vi "Vision Research Phantom Series PhLV Progress.vi"(3 "Continue":bool, 5 "Error In (no error)":errorcluster, 7 "CallID":u32) -> (16 "pPercent":u32, 19 "Error Out":errorcluster)   [LabVIEW 2013, in "VRI.lvlib"]
doc: "PhCon.dll\n\nUse this to have a progress indicator (ex. when reading the stg from flash or saving a cine)\n\nPhLVProgress\nHRESULT PhLVProgress(UINT CallID, PUINT pPercent, BOOL Continue);\n\nParameters Description\nCallID (in) The call identifier (a number from 1 to 15), which was passed as a \n PROGRESSCALLBACK parameter in a time consuming function.\npPercent(out) The percentage of work done for the time consuming routine call, identified\n by CallID. \nContinue(in) Specifies if the function must continue.\n TRUE - to continue\n FALSE - to stop the function call, and force it to return.\nReturn HRESULT (0 = Ok)\nComments This function is used as a progress indicator for time-consuming functions.\n It is designed to work with environments which do not support function\n pointers (like LabVIEW).\n The time-consuming function call and the PhLVProgress call must be in \n different threads.\n In LabVIEW the time-consuming function call node must be set to Reentrant.\n All API calls that have a PROGRESSCALLBACK function pointer parameter\n accept a CallID in it. CallID is a UINT and it must be in the range [1, 15]. \n After calling such a function, you can call PhLVProgress from another thread\n to see the amount of work done or to stop the operation. \n\nWritten by:\nBLOOMY CONTROLS, INC\nWINDSOR, CT 06095, USA\n860-298-9925\nwww.bloomy.com\nV1.0.0\nMay, 2004"
uses:
  VRI.lvlib
  Phantom DLLs/PhCon.Dll
panel:
  # "For instructions on the use of this VI, press Ctrl+H to display the help window and move the mouse over the icon, controls, and indicators"
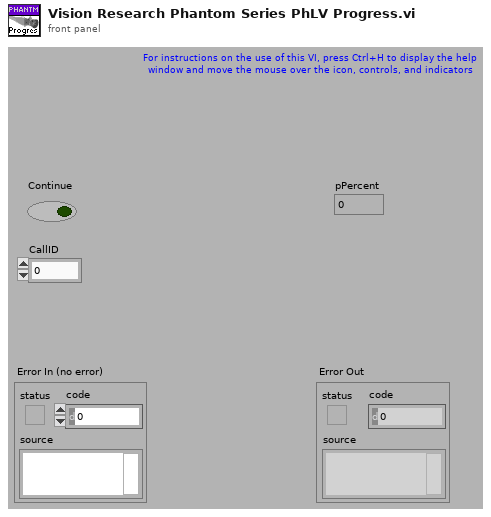
[diagram p1: front panel]
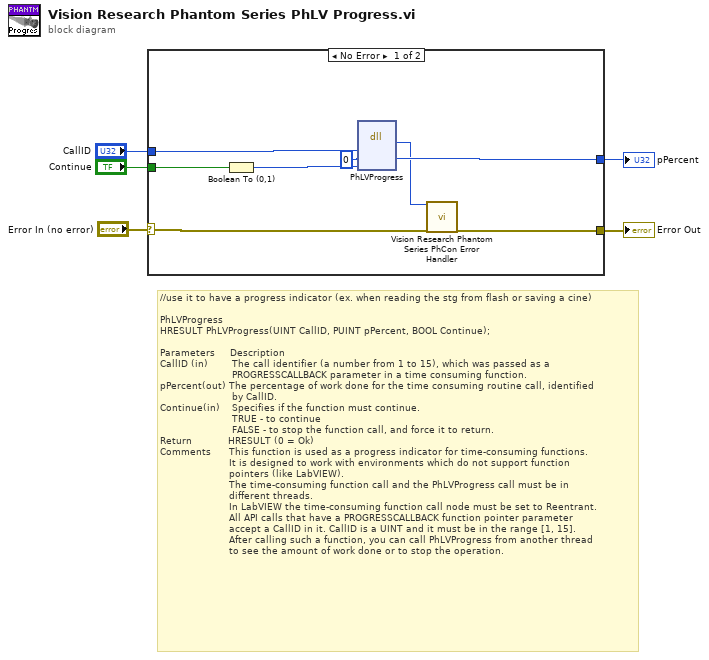
[diagram p0: block diagram]
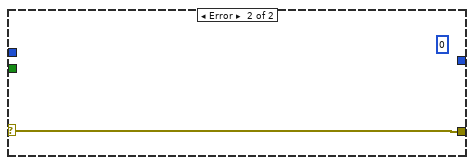
[diagram p2: hidden frame]
diagram:
  # "//use it to have a progress indicator (ex. when reading the stg from flash or saving a cine)\n\nPhLVProgress\nHRESULT PhLVProgress(UINT CallID, PUINT pPercent, BOOL Continue);\n\nParameters     Description\nCallID (in)        The call identifier (a number from 1 to 15), which was passed as a \n                        PROGRESSCALLBACK parameter in a time consuming function.\npPercent(out) The percentage of work done for the time consuming routine call, identified\n                        by CallID. \nContinue(in)    Specifies if the function must continue.\n                        TRUE - to continue\n                        FALSE - to stop the function call, and force it to return.\nReturn            HRESULT (0 = Ok)\nComments      This function is used as a progress indicator for time-consuming functions.\n                       It is designed to work with environments which do not support function\n                       pointers (like LabVIEW).\n                       The time-consuming function call and the PhLVProgress call must be in \n                       different threads.\n                       In LabVIEW the time-consuming function call node must be set to Reentrant.\n                       All API calls that have a PROGRESSCALLBACK function pointer parameter\n                       accept a CallID in it. CallID is a UINT and it must be in the range [1, 15]. \n                       After calling such a function, you can call PhLVProgress from another thread\n                       to see the amount of work done or to stop the operation."
  n1 = case shown="No Error" "Error In (no error)" {
    selector: "Error In (no error)" -> [w13 w14]
    tunnel: [w12 w14] -> w4
    tunnel: "Continue" -> [w11 _]
    tunnel: "CallID" -> [w10 _]
    tunnel: [w9 _] -> w1
    frame No Error {
      n2 = Boolean To (0,1)(Boolean=w11) -> (0, 1=w6:i16)
      n3 = dll-call lib="C:/Projects/SDK/64-bit/Vision Research Phantom Series Labview Driver/Phantom DLLs/PhCon.dll" fn="PhLVProgress"("CallID"=w10, "pPercent"=u32 0, "Continue"=w6) -> ("HRESULT"=w8:u32, "pPercent"=w9:u32)  [unwired: 4 in, 3 out]
      n4 = call "Vision Research Phantom Series PhCon Error Handler.vi"("ErrNo"=w8, "Error In (no error)"=w13) -> ("Error Out"=w12:errorcluster)  [unwired: 17 out]
    }
    frame Error {
      (unwired) 0
    }
  }
  "Error Out" <- w4
  "pPercent" <- w1
